vi "Print PDF.vi"(5 "Print (T)":bool=TRUE, 6 "error in (no error)":errorcluster, 9 "path":path) -> (0 "error out":errorcluster)   [LabVIEW 2019, in "Exaprom PDF.lvlib"]
doc: "Prints the PDF report.\n\n<B>FRANÇAIS</B>\nImprime le rapport PDF.\n\nVersion 1.0\nDeveloped by Jean-Marc Simard\nCopyright © 2010, Exaprom Inc.\nAll rights reserved.\nLicense: BSD"
uses:
  Exaprom PDF.lvlib
panel:
  in  "PDF to print":refnum<k7>(container)
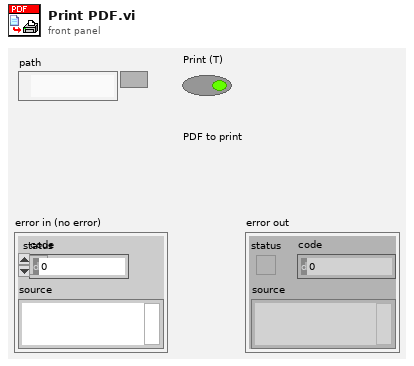
[diagram p1: front panel]
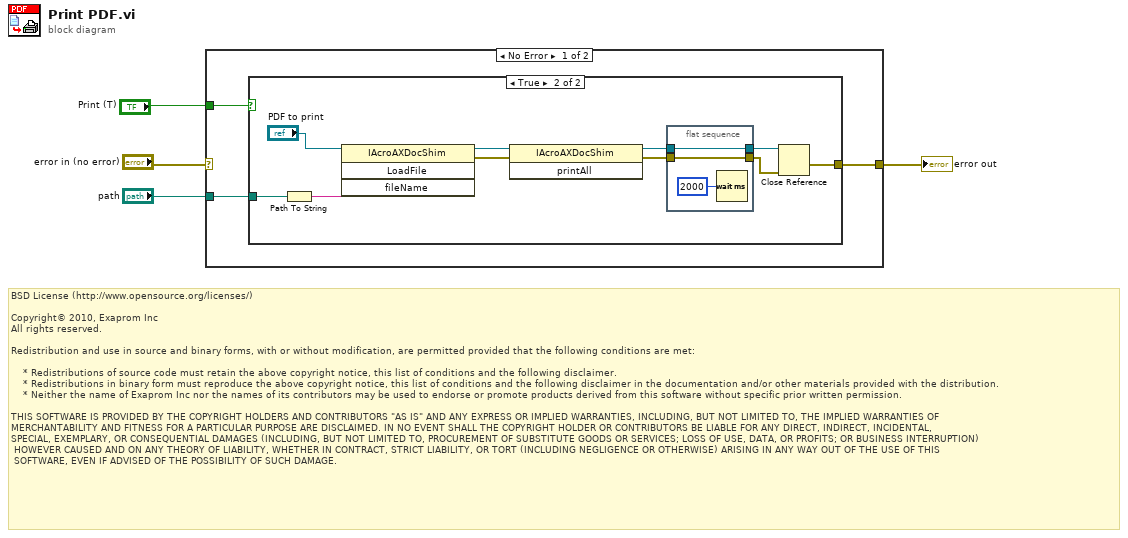
[diagram p0: block diagram]
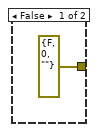
[diagram p2: hidden frame]
diagram:
  # "BSD License (http://www.opensource.org/licenses/)\n\nCopyright© 2010, Exaprom Inc\nAll rights reserved.\n\nRedistribution and use in source and binary forms, with or without modification, are permitted provided that the following conditions are met:\n\n    * Redistributions of source code must retain the above copyright notice, this list of conditions and the following disclaimer.\n    * Redistributions in binary form must reproduce the above copyright notice, this list of conditions and the following disclaimer in the documentation and/or other materials provided with the distribution.\n    * Neither the name of Exaprom Inc nor the names of its contributors may be used to endorse or promote products derived from this software without specific prior written permission.\n\nTHIS SOFTWARE IS PROVIDED BY THE COPYRIGHT HOLDERS AND CONTRIBUTORS \"AS IS\" AND ANY EXPRESS OR IMPLIED WARRANTIES, INCLUDING, BUT NOT LIMITED TO, THE IMPLIED WARRANTIES OF \nMERCHANTABILITY AND FITNESS FOR A PARTICULAR PURPOSE ARE DISCLAIMED. IN NO EVENT SHALL THE COPYRIGHT HOLDER OR CONTRIBUTORS BE LIABLE FOR ANY DIRECT, INDIRECT, INCIDENTAL,\nSPECIAL, EXEMPLARY, OR CONSEQUENTIAL DAMAGES (INCLUDING, BUT NOT LIMITED TO, PROCUREMENT OF SUBSTITUTE GOODS OR SERVICES; LOSS OF USE, DATA, OR PROFITS; OR BUSINESS INTERRUPTION)\n HOWEVER CAUSED AND ON ANY THEORY OF LIABILITY, WHETHER IN CONTRACT, STRICT LIABILITY, OR TORT (INCLUDING NEGLIGENCE OR OTHERWISE) ARISING IN ANY WAY OUT OF THE USE OF THIS\n SOFTWARE, EVEN IF ADVISED OF THE POSSIBILITY OF SUCH DAMAGE."
  n1 = case shown="No Error" "error in (no error)" {
    selector: "error in (no error)" -> [_ w22]
    tunnel: [w7 w22] -> w2
    tunnel: "path" -> [w6 _]
    tunnel: "Print (T)" -> [w5 _]
    frame No Error {
      n2 = case shown="True" w5 {
        tunnel: [errorcluster {"status"=FALSE, "code"=0, "source"=""} ("error out") w11] -> w7
        tunnel: w6 -> [_ w9]
        frame False {
        }
        frame True {
          n3 = Path To String(path=w9) -> (string=w10:string)
          n4 = invoke class="IAcroAXDocShim" method="LoadFile"(reference="PDF to print", "fileName"=w10) -> (reference out=w17:refnum<k7>, error out=w16:errorcluster)  [unwired: 2 in, 2 out]
          n5 = invoke class="IAcroAXDocShim" method="printAll"(reference=w17, error in=w16) -> (reference out=w12:refnum<k7>, error out=w15:errorcluster)  [unwired: 1 in, 1 out]
          n6 = flat-sequence {
            tunnel: w15 -> [w20]
            tunnel: [w20] -> w14
            tunnel: [w19] -> w13
            tunnel: w12 -> [w19]
            frame #0 {
              n7 = Wait (ms)(milliseconds to wait=u32 2000) -> ()  [unwired: 1 out]
            }
          }
          n8 = Close Reference(reference=w13, error in (no error)=w14) -> (error out=w11:errorcluster)
        }
      }
    }
    frame Error {
    }
  }
  "error out" <- w2
